vi "DAQmxBuildTasks.vi"(10 "Device port info":T1[](array[typedef]), 11 "taskNamesIn":string[](array[string])) -> (0 "error out":errorcluster, 2 "FsOut":dbl[](array[numeric]))   [LabVIEW 2022 SP3]
uses:
  Device ID port info.ctl
  f383c325-543f-44f0-b992-ec9ac167a994.vi
  <vilib>/DAQmx/create/channels.llb/DAQmx Create Channel (AI-Voltage-Custom with Excitation).vi
  <vilib>/DAQmx/create/channels.llb/DAQmx Create Channel (AI-Voltage-Basic).vi
  <vilib>/DAQmx/configure/timing.llb/DAQmx Timing (Sample Clock).vi
  <resource>/objmgr/daqmx.rc
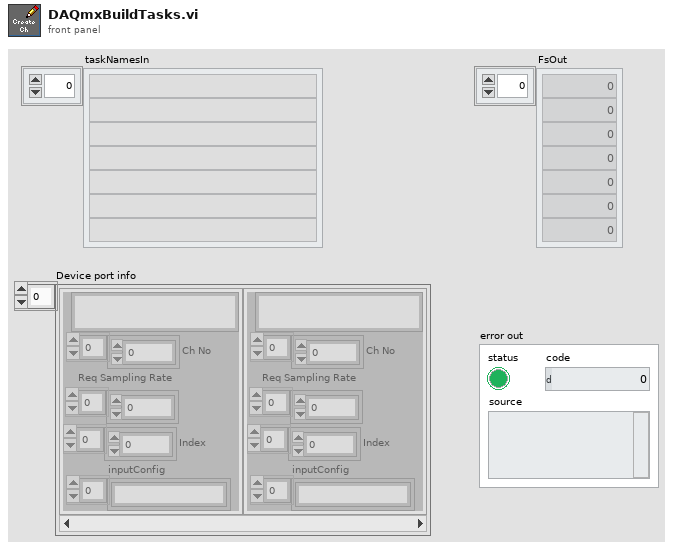
[diagram p1: front panel]
types:
  T1 = typedef "Device ID port info.ctl" = cluster{"Ch No":i16[], "Req Sampling Rate":dbl[], "Port":string, "Index":i32[], "inputConfig":string[]}
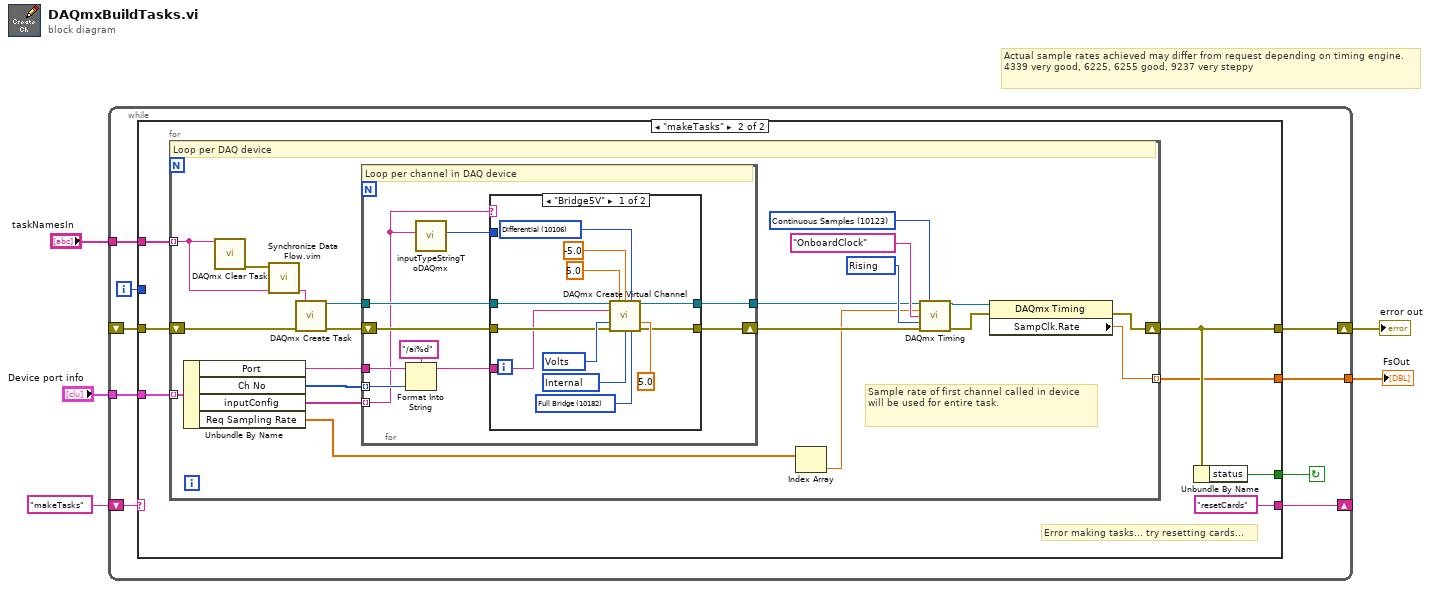
[diagram p0: block diagram]
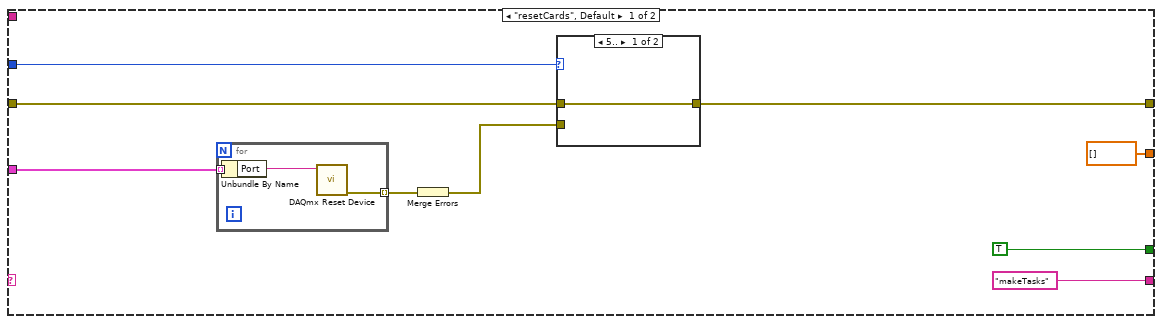
[diagram p2: hidden frame]
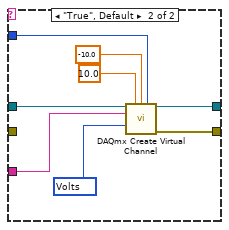
[diagram p4: hidden frame]
diagram:
  # "Actual sample rates achieved may differ from request depending on timing engine. 4339 very good, 6225, 6255 good, 9237 very steppy"
  n1 = while {
    tunnel: "Device port info" -> [w14]
    shift-right: [w11] -> _
    shift-left: "makeTasks" -> [w12]
    shift-right: [w9] -> w3
    shift-left: _ -> [w8]
    tunnel: "taskNamesIn" -> [w7]
    tunnel: [w6] -> w1
    i -> [w10]
    stop <- w13 continue-if-true
    n2 = case shown="\"makeTasks\"" w12 {
      tunnel: w14 -> [w20 w35]
      tunnel: [TRUE w33] -> w13
      tunnel: ["makeTasks" "resetCards"] -> w11
      tunnel: w10 -> [w21 _]
      tunnel: [w17 w32] -> w9
      tunnel: w8 -> [w16 w31]
      tunnel: w7 -> [_ w30]
      tunnel: [dbl[] [] w29] -> w6
      frame "resetCards", Default {
        n3 = for {
          tunnel: w20 -> [w26] mode=indexing
          tunnel: [w24] -> w19 mode=indexing
          n4 = Unbundle By Name(w26) -> ("Port"=w25:string)
          n5 = call <vilib>:"DAQmx Reset Device.vi"("device in"=w25) -> ("error out"=w24:errorcluster)  [unwired: 14 in]
        }
        n6 = Merge Errors(w19) -> (w18:errorcluster)
        n7 = case shown="5.." w21 {
          tunnel: [w27 w28] -> w17
          tunnel: w18 -> [_ w28]
          tunnel: w16 -> [w27 _]
          frame 5.. {
          }
          frame 0, Default {
          }
        }
      }
      frame "makeTasks" {
        # "Error making tasks... try resetting cards..."
        n8 = for {
          tunnel: w35 -> [w55] mode=indexing
          shift-right: [w37] -> w32
          shift-left: w31 -> [w56]
          tunnel: w30 -> [w43] mode=indexing
          tunnel: [w36] -> w29 mode=indexing
          w50 = 10280 items=["Rising"=10280, "Falling"=10171] ("active edge")
          w52 = 10123 items=["Finite Samples"=10178, "Continuous Samples"=10123, "Hardware Timed Single Point"=12522] ("sample mode")
          # "Sample rate of first channel called in device will be used for entire task."
          # "Loop per DAQ device"
          n9 = Unbundle By Name(w55) -> ("Port"=w46:string, "Ch No"=w47:i16[], "inputConfig"=w42:string[], "Req Sampling Rate"=w41:dbl[])
          n10 = call <vilib>:"DAQmx Clear Task.vi"("task in"=w43) -> ("error out"=w45:errorcluster)  [unwired: 14 in]
          n11 = call "Synchronize Data Flow.vim"("input 4"=w43, "input 1"=w45) -> ("output 4"=w44:string)  [unwired: 2 in, 3 out]
          n12 = call <vilib>:"DAQmx Create Task.vi"("new task name"=w44, "error in"=w56) -> ("task out"=w54:refnum<k21>, "error out"=w53:errorcluster)  [unwired: 3 in, 9 out]
          n13 = for {
            shift-right: [w61] -> w48
            shift-left: w53 -> [w64]
            tunnel: w46 -> [w60]
            tunnel: w47 -> [w59] mode=indexing
            tunnel: w54 -> [w65]
            tunnel: [w62] -> w49
            tunnel: w42 -> [w58] mode=indexing
            # "Loop per channel in DAQ device"
            n14 = Format Into String(format string="/ai%d", initial string=w60, w59) -> (resulting string=w63:string)  [unwired: 1 in, 1 out]
            n15 = call "inputTypeStringToDAQmx.vi"("inputConfig"=w58) -> ("input terminal configuration"=w57:i32)  [unwired: 10 in]
            n16 = case shown="\"Bridge5V\"" w58 {
              tunnel: w65 -> [w78 w81]
              tunnel: w64 -> [w73 _]
              tunnel: w63 -> [w69 w80]
              tunnel: [w68 w83] -> w62
              tunnel: [w67 w82] -> w61
              tunnel: w57 -> [_ w79]
              frame "Bridge5V" {
                w71 = 10182 items=["Full Bridge"=10182, "Half Bridge"=10187, "Quarter Bridge"=10270, "No Bridge"=10228] ("bridge configuration")
                w72 = 10200 items=["Internal"=10200, "External"=10167, "None"=10230] ("voltage excitation source")
                w74 = 10348 items=["Volts"=10348, "From Custom Scale"=10065] ("units")
                w77 = 10106 items=["Default"=-1, "RSE"=10083, "NRSE"=10078, "Differential"=10106, "Pseudodifferential"=12529] ("input terminal configuration")
                n17 = call-poly <vilib>:"DAQmx Create Virtual Channel.vi"("task in"=w78, "maximum value"=5.0, "minimum value"=-5.0, "input terminal configuration"=w77, "physical channels"=w69, "units"=w74, "voltage excitation value"=5.0, "error in"=w73, "voltage excitation source"=w72, "bridge configuration"=w71) -> ("task out"=w68:refnum<k21>, "error out"=w67:errorcluster)  [unwired: 3 in, 1 out]
              }
              frame "True", Default {
                w84 = 10348 items=["Volts"=10348, "From Custom Scale"=10065] ("units")
                n18 = call-poly <vilib>:"DAQmx Create Virtual Channel.vi"("task in"=w81, "maximum value"=10.0, "minimum value"=-10.0, "input terminal configuration"=w79, "physical channels"=w80, "units"=w84) -> ("task out"=w83:refnum<k21>, "error out"=w82:errorcluster)  [unwired: 3 in, 5 out]
              }
            }
          }
          n19 = Index Array(array=w41) -> (element=w40:dbl)  [unwired: 1 in]
          n20 = call-poly <vilib>:"DAQmx Timing.vi"("task/channels in"=w49, "sample mode"=w52, "rate"=w40, "source"=tag "OnboardClock", "active edge"=w50, "error in"=w48) -> ("task out"=w39:refnum<k21>, "error out"=w38:errorcluster)  [unwired: 1 in, 7 out]
          n21 = property class="DAQmx Timing"(reference=w39, error in=w38) -> (error out=w37:errorcluster, "SampClk.Rate"=w36:dbl)  [unwired: 1 out]
        }
        n22 = Unbundle By Name(w32) -> ("status"=w33:bool)
      }
    }
  }
  "error out" <- w3
  "FsOut" <- w1
